vi "New.vi"(4 "Properties":T2={"Background Color"=2147483647, "Axis Background"=2147483647, "Left Margin"=nan, "Right Margin"=nan, "Bottom Margin"=nan, "Top Margin"=nan, "Aspect Ratio"=nan} {"Axis Background" items=["Automatic"=2147483647, "Black"=0, "White"=16777215, "Red"=16711680, "Green"=2263842, "Blue"=255, "Cyan"=65535, "Magenta"=16711935, "Yellow"=16776960]; "Background Color" items=["Automatic"=2147483647, "Black"=0, "White"=16777215, "Red"=16711680, "Green"=2263842, "Blue"=255, "Cyan"=65535, "Magenta"=16711935, "Yellow"=16776960]}, 5 "Y Axis Scale":T1, 7 "X Axis Scale":T1, 8 "error in (no error)":errorcluster, 10 "Plot Type":T4) -> (0 "error out":errorcluster, 3 "Plot ID":T5 format="%x")   [LabVIEW 2013, in "Advanced Plotting Toolkit.lvlib"]
doc: "Create a new plot, returning a plot identifier. You must eventually close the identifier (see Close.vi) to avoid resource leaks."
uses:
  Advanced Plotting Toolkit.lvlib
  typedefs/PlotID.ctl
  NewPlotType.ctl
  NewPlotProperties.ctl
  typedefs/PlotColor.ctl
  NewPlotScales.ctl
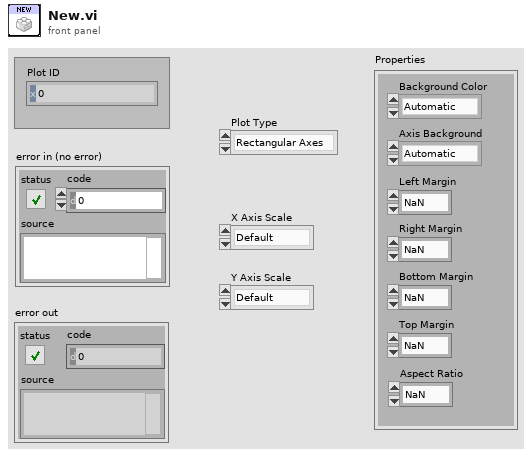
[diagram p1: front panel]
types:
  T1 = typedef "Advanced Plotting Toolkit.lvlib/NewPlotScales.ctl" = enum16{"Default", "Linear", "Log", "Symlog"}
  T2 = typedef "Advanced Plotting Toolkit.lvlib/NewPlotProperties.ctl" = cluster{"Background Color":T3, "Axis Background":T3, "Left Margin":dbl, "Right Margin":dbl, "Bottom Margin":dbl, "Top Margin":dbl, "Aspect Ratio":dbl}
  T3 = typedef "Advanced Plotting Toolkit.lvlib/PlotColor.ctl" = u32
  T4 = typedef "Advanced Plotting Toolkit.lvlib/NewPlotType.ctl" = enum16{"Rectangular Axes", "Polar Axes"}
  T5 = typedef "Advanced Plotting Toolkit.lvlib/PlotID.ctl" = i32
  T6 = typedef "Advanced Plotting Toolkit.lvlib/KeyValue.ctl" = cluster{"Key":string, "Value":string}
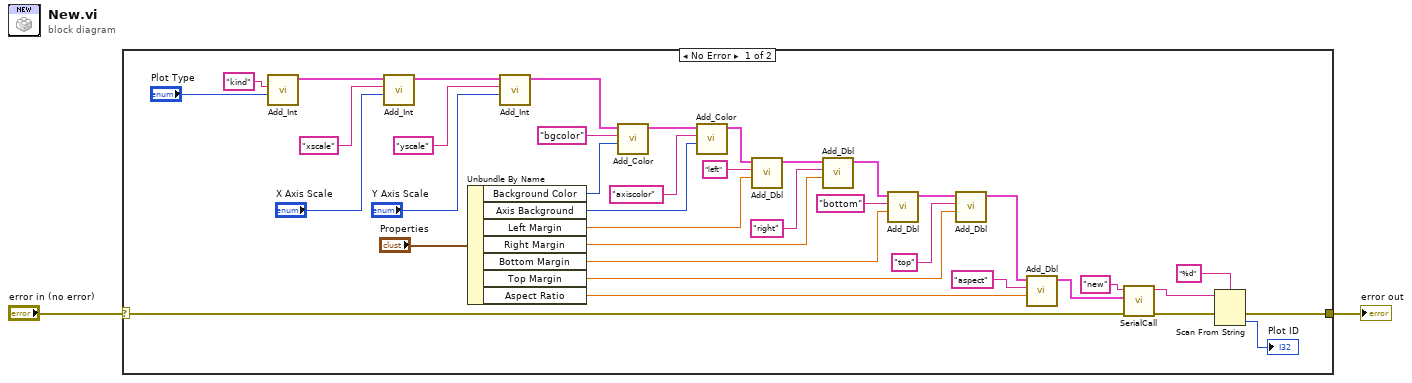
[diagram p0: block diagram]
diagram:
  n1 = case shown="No Error" "error in (no error)" {
    selector: "error in (no error)" -> [w39 w41]
    tunnel: [w33 w41] -> w2
    frame No Error {
      n2 = call "Add_Int.vi"("Value"="Plot Type", "Key"="kind") -> ("Keyword Array Out"=w9:T6[])  [unwired: 9 in]
      n3 = call "Add_Int.vi"("Value"="X Axis Scale", "Key"="xscale", "Keyword Array"=w9) -> ("Keyword Array Out"=w5:T6[])  [unwired: 8 in]
      n4 = Unbundle By Name("Properties") -> ("Background Color"=w15:T3, "Axis Background"=w17:T3, "Left Margin"=w24:dbl, "Right Margin"=w23:dbl, "Bottom Margin"=w22:dbl, "Top Margin"=w21:dbl, "Aspect Ratio"=w11:dbl)
      n5 = call "Add_Int.vi"("Value"="Y Axis Scale", "Key"="yscale", "Keyword Array"=w5) -> ("Keyword Array Out"=w4:T6[])  [unwired: 8 in]
      n6 = call "Add_Color.vi"("Color"=w15, "Key"="bgcolor", "Keyword Array"=w4) -> ("Keyword Array Out"=w14:T6[])  [unwired: 8 in]
      n7 = call "Add_Color.vi"("Color"=w17, "Key"="axiscolor", "Keyword Array"=w14) -> ("Keyword Array Out"=w19:T6[])  [unwired: 8 in]
      n8 = call "Add_Dbl.vi"("Value"=w24, "Key"="left", "Keyword Array"=w19) -> ("Keyword Array Out"=w25:T6[])  [unwired: 8 in]
      n9 = call "Add_Dbl.vi"("Value"=w23, "Key"="right", "Keyword Array"=w25) -> ("Keyword Array Out"=w26:T6[])  [unwired: 8 in]
      n10 = call "Add_Dbl.vi"("Value"=w22, "Key"="bottom", "Keyword Array"=w26) -> ("Keyword Array Out"=w20:T6[])  [unwired: 8 in]
      n11 = call "Add_Dbl.vi"("Value"=w21, "Key"="top", "Keyword Array"=w20) -> ("Keyword Array Out"=w13:T6[])  [unwired: 8 in]
      n12 = call "Add_Dbl.vi"("Value"=w11, "Key"="aspect", "Keyword Array"=w13) -> ("Keyword Array Out"=w12:T6[])  [unwired: 8 in]
      n13 = call "SerialCall.vi"("error in (no error)"=w39, "data"=w12, "Resource"="new") -> ("error out"=w36:errorcluster, "Response"=w35:string)  [unwired: 7 in]
      n14 = Scan From String(format string="%d", input string=w35, error in=w36) -> (error out=w33:errorcluster, output 1=→"Plot ID":T5)  [unwired: 2 in, 2 out]
    }
    frame Error {
    }
  }
  "error out" <- w2
